vi "Update UI Control value.vi"(10 "Boolean":bool, 11 "Array":refnum<vi>[](array[refnum])) -> ()   [LabVIEW 2016, in "Settings Editor.lvlib"]
uses:
  Settings Editor.lvlib
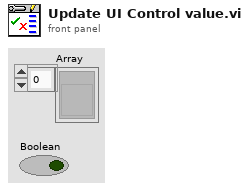
[diagram p1: front panel]
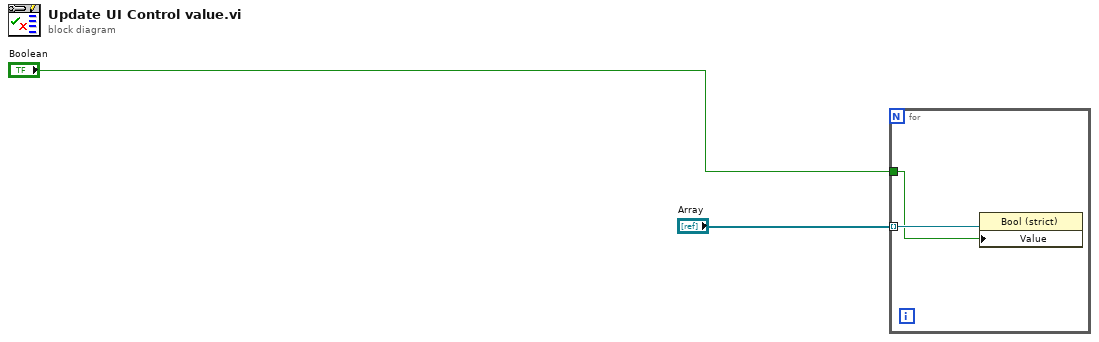
[diagram p0: block diagram]
diagram:
  n1 = for {
    tunnel: "Array" -> [w4] mode=indexing
    tunnel: "Boolean" -> [w3]
    n2 = property class="Bool (strict)"(reference=w4, "Value"=w3) -> ()  [unwired: 1 in, 2 out]
  }
